vi "einzel.vi"() -> ()   [LabVIEW 2013]
panel:
  out "Return Values":string[](array[string])
  out "appended array":string[](array[string])
  in  "stop":bool
  out "V_needle":dbl
  out "V_pelletron":dbl
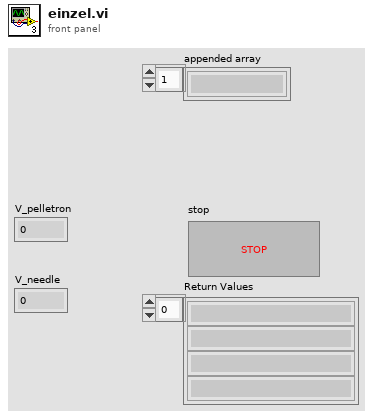
[diagram p1: front panel]
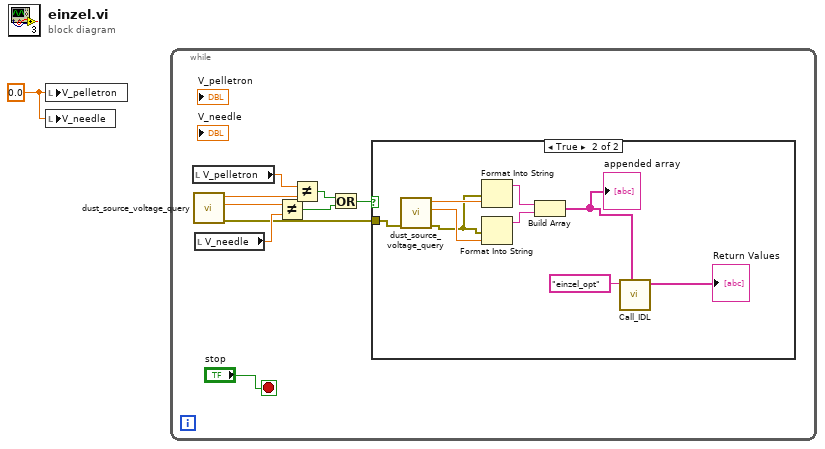
[diagram p0: block diagram]
diagram:
  w1 = 0.0 ("V_pelletron")
  n1 = local write "V_pelletron"(w1) -> ()
  n2 = local write "V_needle"(w1) -> ()
  n3 = while {
    stop <- "stop" stop-if-true
    n4 = local read "V_pelletron"() -> (w6:dbl)
    n5 = call "dust_source_voltage_query.vi"() -> ("error out"=w2:errorcluster, "needle_voltage"=w9:dbl, "high_voltage"=w7:dbl)  [unwired: 9 in]
    n6 = local read "V_needle"() -> (w8:dbl)
    n7 = Not Equal?(x=w9, y=w8) -> (x != y?=w4:bool)
    n8 = Not Equal?(x=w6, y=w7) -> (x != y?=w5:bool)
    n9 = Or(x=w5, y=w4) -> (x .or. y?=w3:bool)
    n10 = case shown="True" w3 {
      tunnel: w2 -> [_ w18]
      frame False {
      }
      frame True {
        n11 = call "dust_source_voltage_query.vi"("error in (no error)"=w18) -> ("error out"=w15:errorcluster, "needle_voltage"=w16:dbl, "high_voltage"=w17:dbl)  [unwired: 8 in]
        n12 = Format Into String(error in=w15, w17) -> (resulting string=w14:string)  [unwired: 2 in, 1 out]
        n13 = Format Into String(error in=w15, w16) -> (resulting string=w13:string)  [unwired: 2 in, 1 out]
        n14 = Build Array(w14, w13) -> (w12:string[])
        "appended array" <- w12
        n15 = call "Call_IDL.vi"("Arguments"=w12, "IDL function"="einzel_opt") -> ("Return Values"=→"Return Values":string[])  [unwired: 5 in, 4 out]
      }
    }
  }
